vi "Frequency_sweep_measureXandY_w_2w_3w_MFLI_PK_v4.0.vi"() -> ()   [LabVIEW 2016]
uses:
  Labview Drivers/MFLI/LabOneLabVIEW-22.02.26577/LabOneLabVIEW-22.02.26577/Zurich Instruments LabOne/Public/Data/ziTypeDemodSampleSingle.ctl
  Labview Drivers/MFLI/LabOneLabVIEW-22.02.26577/LabOneLabVIEW-22.02.26577/Zurich Instruments LabOne/Public/Configure/ziSetValueDouble.vi
  Labview Drivers/MFLI/LabOneLabVIEW-22.02.26577/LabOneLabVIEW-22.02.26577/Zurich Instruments LabOne/Public/Configure/ziGetValueDemodSampleEx.vi
  Labview Drivers/MFLI/LabOneLabVIEW-22.02.26577/LabOneLabVIEW-22.02.26577/Zurich Instruments LabOne/Zurich Instruments LabOne.lvlib
panel:
  in  "Tab Control":T1(tab)=enum."Vy"
  out "Vx_w vs  Frequency":cluster{dbl, "Field Reading":dbl}[](graph)=[{2.1337108522522826e-07, "Field Reading"=1.0007121497539348e-06}, {2.0018204953851064e-08, "Field Reading"=1.0969598663661376e-07}, {3.474074033482476e-08, "Field Reading"=1.9016075130631681e-07}, {5.6400419155691035e-08, "Field Reading"=2.706780203266455e-07}, {7.134741663483111e-08, "Field Reading"=3.625194153695155e-07}, {8.711957733763268e-08, "Field Reading"=4.6186456260881066e-07}, {1.039613386460647e-07, "Field Reading"=5.541771498802743e-07}, {1.290159481540569e-07, "Field Reading"=6.517488283090827e-07}, {1.442006622421336e-07, "Field Reading"=7.441421685111633e-07}, {1.6579779771841864e-07, "Field Reading"=8.4200282004452e-07}, {1.7667431320194624e-07, "Field Reading"=9.371894272094692e-07}, {2.0346799660082097e-07, "Field Reading"=1.0346819690568719e-06}, {2.1275449478314156e-07, "Field Reading"=1.1273455634288892e-06}, {2.2792303722372882e-07, "Field Reading"=1.2246113813938451e-06}, {2.506226161778463e-07, "Field Reading"=1.3169699353558023e-06}, {2.6686786096204173e-07, "Field Reading"=1.4106741902497636e-06}, {2.979630377408132e-07, "Field Reading"=1.5068897992871093e-06}, {3.1162936250255217e-07, "Field Reading"=1.6013785409354697e-06}, {3.2854904168138843e-07, "Field Reading"=1.7007967107121696e-06}, {3.4501678279448686e-07, "Field Reading"=1.7932741209540488e-06}, {3.5732655253185603e-07, "Field Reading"=1.891133061059139e-06}, {3.7678513716337806e-07, "Field Reading"=1.9837632139333797e-06}, {3.8857693765173823e-07, "Field Reading"=2.078638757139878e-06}, {4.070455630330932e-07, "Field Reading"=2.1777621608691614e-06}, {4.3651006057087547e-07, "Field Reading"=2.270487653250022e-06}, {4.535609885287045e-07, "Field Reading"=2.364817703267964e-06}, {4.800092323465329e-07, "Field Reading"=2.4630513126122318e-06}, {4.872172260420143e-07, "Field Reading"=2.560612214294704e-06}, {5.029105394973937e-07, "Field Reading"=2.653407522930296e-06}, {5.207137968885614e-07, "Field Reading"=2.7508846993110185e-06}, {5.449974912672081e-07, "Field Reading"=2.8437164663468094e-06}, {5.549097834910874e-07, "Field Reading"=2.941117576580943e-06}, {5.789147944756835e-07, "Field Reading"=3.0334756142859178e-06}, {5.940331669154695e-07, "Field Reading"=3.130923358288321e-06}, {6.192662248173834e-07, "Field Reading"=3.223457045619671e-06}, {6.338859460756282e-07, "Field Reading"=3.3210140787077685e-06}, {6.617730672082958e-07, "Field Reading"=3.4134337904467758e-06}, {6.708744764433933e-07, "Field Reading"=3.511218639909905e-06}, {6.876034184888421e-07, "Field Reading"=3.6064791588715936e-06}, {7.081705825683568e-07, "Field Reading"=3.704194984998823e-06}, {7.341349902267621e-07, "Field Reading"=3.796795088130521e-06}, {7.500412173627324e-07, "Field Reading"=3.894221622472711e-06}, {7.635282212201655e-07, "Field Reading"=3.986359362120525e-06}, {7.839559208505005e-07, "Field Reading"=4.084105589459172e-06}, {7.991337007295971e-07, "Field Reading"=4.176440151889332e-06}, {8.175550663233945e-07, "Field Reading"=4.274041338897146e-06}, {8.360511976155764e-07, "Field Reading"=4.366718612721536e-06}, {8.595654269642977e-07, "Field Reading"=4.46481586459238e-06}, {8.846044621269243e-07, "Field Reading"=4.559710869350914e-06}, {8.902214589762566e-07, "Field Reading"=4.6535858762473605e-06}, {9.13930972707384e-07, "Field Reading"=4.751211544539011e-06}, {9.218629476317926e-07, "Field Reading"=4.843674806906942e-06}, {9.389346568153207e-07, "Field Reading"=4.94148963023105e-06}, {9.661788530141893e-07, "Field Reading"=5.0340339305698605e-06}, {9.734275114489362e-07, "Field Reading"=5.134274890899915e-06}, {9.91273930192609e-07, "Field Reading"=5.227194198108034e-06}, {1.0062090937222443e-06, "Field Reading"=5.324543514118811e-06}, {1.0324830232331714e-06, "Field Reading"=5.417068558459935e-06}, {1.0500453704719826e-06, "Field Reading"=5.514414049876445e-06}, {1.0818020141498576e-06, "Field Reading"=5.606738838727315e-06}, {1.0919981214621985e-06, "Field Reading"=5.943499955969014e-06}, {1.1041062115858416e-06, "Field Reading"=5.802825671371831e-06}, {1.12928896400331e-06, "Field Reading"=5.8897635364887065e-06}, {1.1492595887607054e-06, "Field Reading"=5.986959246668246e-06}, {1.1525838773614565e-06, "Field Reading"=6.079112281920131e-06}, {1.1732006667255544e-06, "Field Reading"=6.176765549637453e-06}, {1.193444625294635e-06, "Field Reading"=6.2693583656248445e-06}, {1.2101538188023656e-06, "Field Reading"=6.369277338631168e-06}, {1.2318147585414787e-06, "Field Reading"=6.462177680852612e-06}, {1.2413491771177379e-06, "Field Reading"=6.554239754143973e-06}, {1.2731631837142253e-06, "Field Reading"=6.653541226069562e-06}, {1.2825564782833625e-06, "Field Reading"=6.7454110623267924e-06}, {1.2992348301055137e-06, "Field Reading"=6.843115368447837e-06}, {1.316693256967963e-06, "Field Reading"=6.935702965257668e-06}, {1.343852132299077e-06, "Field Reading"=7.033596304342718e-06}, {0.0003223256295561193, "Field Reading"=7.130369502789653e-06}, {0.0010682796466779994, "Field Reading"=7.237712618778445e-06}, {0.0011012721847992696, "Field Reading"=7.315133567183911e-06}, {0.0011336841810168491, "Field Reading"=7.4123545054478695e-06}, {0.0011614058556892847, "Field Reading"=7.504304430827025e-06}, {0.001182885890671154, "Field Reading"=7.602366955750201e-06}, {0.001200897535521615, "Field Reading"=7.69976061587441e-06}, {0.00121594401470624, "Field Reading"=7.792677109208386e-06}, {0.0012308027651267619, "Field Reading"=7.886128685028496e-06}, {0.0012456418637471253, "Field Reading"=7.983615236672288e-06}, {0.001257564969772003, "Field Reading"=8.075760842161778e-06}, {0.0012690336996615858, "Field Reading"=8.170723157183957e-06}, {0.0012814644345765262, "Field Reading"=8.268995175290895e-06}, {0.0012910253378675095, "Field Reading"=8.363131378141633e-06}, {0.001301444806581894, "Field Reading"=8.45644533427298e-06}, {0.0013106148752890106, "Field Reading"=8.551458283635111e-06}, {0.0013201336522581891, "Field Reading"=8.65161959339898e-06}, {0.0013282012490195363, "Field Reading"=8.74416723601607e-06}, {0.0013370451945670784, "Field Reading"=8.841765835802203e-06}, {0.001345475691336453, "Field Reading"=8.933978266213217e-06}, {0.0013541642420234728, "Field Reading"=9.031643266856203e-06}, {0.0013602243952778926, "Field Reading"=9.123705087732138e-06}, {0.0013678078924535615, "Field Reading"=9.221510724442928e-06}, {0.0013749931650039048, "Field Reading"=9.319154251910434e-06}, {0.0013817418853904447, "Field Reading"=9.409423170522308e-06}, {0.0013877620940512577, "Field Reading"=9.50720467327743e-06}, {0.0013893900209027232, "Field Reading"=9.522740574798281e-06}, {0.0013841293323999348, "Field Reading"=9.444358568387913e-06}, {0.0013770955503089543, "Field Reading"=9.34786117205707e-06}, {0.0013707463881856257, "Field Reading"=9.255459479065146e-06}, {0.0013638010752030354, "Field Reading"=9.157506360964617e-06}, {0.001356127430849226, "Field Reading"=9.065389480276688e-06}, {0.0013481807501391138, "Field Reading"=8.967105386552946e-06}, {0.0013407950243109453, "Field Reading"=8.872574329619889e-06}, {0.0013327879049762552, "Field Reading"=8.780745564878272e-06}, {0.0013239176518001648, "Field Reading"=8.686977265427215e-06}, {0.0013146578852826479, "Field Reading"=8.586299385882446e-06}, {0.0013048672888862206, "Field Reading"=8.493635331032656e-06}, {0.0012950842712132512, "Field Reading"=8.395823484571033e-06}, {0.0012855051336405129, "Field Reading"=8.303455420153361e-06}, {0.001274818349601112, "Field Reading"=8.209679742685101e-06}, {0.0012618971608759537, "Field Reading"=8.109946125115199e-06}, {0.0012494525821266837, "Field Reading"=8.017364894823338e-06}, {0.001235685913286103, "Field Reading"=7.919657723881713e-06}, {0.0012216877307261714, "Field Reading"=7.824897358413329e-06}, {0.0012037516065472435, "Field Reading"=7.727435253164315e-06}, {0.0011875344677767074, "Field Reading"=7.634970945479442e-06}, {0.0011690885694813937, "Field Reading"=7.537773175917453e-06}, {0.001143867923079635, "Field Reading"=7.445625913634191e-06}, {0.0011139726709101221, "Field Reading"=7.348337041113834e-06}, {0.0010813147907609588, "Field Reading"=7.255852572757193e-06}, {0.0008158901453383064, "Field Reading"=7.15654215348316e-06}, {0.00014586885402730632, "Field Reading"=7.065078532967033e-06}, {6.672313176192101e-06, "Field Reading"=6.97131792702715e-06}, {1.311378694927265e-06, "Field Reading"=6.8592321760864306e-06}, {1.318127585000335e-06, "Field Reading"=6.78165201436255e-06}, {1.2916070805813707e-06, "Field Reading"=6.684382236814962e-06}, {1.2637872492482735e-06, "Field Reading"=6.591615618281428e-06}, {1.2510857193087697e-06, "Field Reading"=6.49373019741343e-06}, {1.2409566576000475e-06, "Field Reading"=6.399307801408899e-06}, {1.215389141425889e-06, "Field Reading"=6.305912312991265e-06}, {1.1948309642776338e-06, "Field Reading"=6.211147873874382e-06}, {1.1729714746286896e-06, "Field Reading"=6.112674813622632e-06}, {1.1526746179431637e-06, "Field Reading"=6.015256707500007e-06}]
  out "Vy_w vs Frequency":cluster{dbl, "Field Reading":dbl}[](graph)=[{2.1337108522522826e-07, "Field Reading"=1.0007121497539348e-06}, {2.0018204953851064e-08, "Field Reading"=1.0969598663661376e-07}, {3.474074033482476e-08, "Field Reading"=1.9016075130631681e-07}, {5.6400419155691035e-08, "Field Reading"=2.706780203266455e-07}, {7.134741663483111e-08, "Field Reading"=3.625194153695155e-07}, {8.711957733763268e-08, "Field Reading"=4.6186456260881066e-07}, {1.039613386460647e-07, "Field Reading"=5.541771498802743e-07}, {1.290159481540569e-07, "Field Reading"=6.517488283090827e-07}, {1.442006622421336e-07, "Field Reading"=7.441421685111633e-07}, {1.6579779771841864e-07, "Field Reading"=8.4200282004452e-07}, {1.7667431320194624e-07, "Field Reading"=9.371894272094692e-07}, {2.0346799660082097e-07, "Field Reading"=1.0346819690568719e-06}, {2.1275449478314156e-07, "Field Reading"=1.1273455634288892e-06}, {2.2792303722372882e-07, "Field Reading"=1.2246113813938451e-06}, {2.506226161778463e-07, "Field Reading"=1.3169699353558023e-06}, {2.6686786096204173e-07, "Field Reading"=1.4106741902497636e-06}, {2.979630377408132e-07, "Field Reading"=1.5068897992871093e-06}, {3.1162936250255217e-07, "Field Reading"=1.6013785409354697e-06}, {3.2854904168138843e-07, "Field Reading"=1.7007967107121696e-06}, {3.4501678279448686e-07, "Field Reading"=1.7932741209540488e-06}, {3.5732655253185603e-07, "Field Reading"=1.891133061059139e-06}, {3.7678513716337806e-07, "Field Reading"=1.9837632139333797e-06}, {3.8857693765173823e-07, "Field Reading"=2.078638757139878e-06}, {4.070455630330932e-07, "Field Reading"=2.1777621608691614e-06}, {4.3651006057087547e-07, "Field Reading"=2.270487653250022e-06}, {4.535609885287045e-07, "Field Reading"=2.364817703267964e-06}, {4.800092323465329e-07, "Field Reading"=2.4630513126122318e-06}, {4.872172260420143e-07, "Field Reading"=2.560612214294704e-06}, {5.029105394973937e-07, "Field Reading"=2.653407522930296e-06}, {5.207137968885614e-07, "Field Reading"=2.7508846993110185e-06}, {5.449974912672081e-07, "Field Reading"=2.8437164663468094e-06}, {5.549097834910874e-07, "Field Reading"=2.941117576580943e-06}, {5.789147944756835e-07, "Field Reading"=3.0334756142859178e-06}, {5.940331669154695e-07, "Field Reading"=3.130923358288321e-06}, {6.192662248173834e-07, "Field Reading"=3.223457045619671e-06}, {6.338859460756282e-07, "Field Reading"=3.3210140787077685e-06}, {6.617730672082958e-07, "Field Reading"=3.4134337904467758e-06}, {6.708744764433933e-07, "Field Reading"=3.511218639909905e-06}, {6.876034184888421e-07, "Field Reading"=3.6064791588715936e-06}, {7.081705825683568e-07, "Field Reading"=3.704194984998823e-06}, {7.341349902267621e-07, "Field Reading"=3.796795088130521e-06}, {7.500412173627324e-07, "Field Reading"=3.894221622472711e-06}, {7.635282212201655e-07, "Field Reading"=3.986359362120525e-06}, {7.839559208505005e-07, "Field Reading"=4.084105589459172e-06}, {7.991337007295971e-07, "Field Reading"=4.176440151889332e-06}, {8.175550663233945e-07, "Field Reading"=4.274041338897146e-06}, {8.360511976155764e-07, "Field Reading"=4.366718612721536e-06}, {8.595654269642977e-07, "Field Reading"=4.46481586459238e-06}, {8.846044621269243e-07, "Field Reading"=4.559710869350914e-06}, {8.902214589762566e-07, "Field Reading"=4.6535858762473605e-06}, {9.13930972707384e-07, "Field Reading"=4.751211544539011e-06}, {9.218629476317926e-07, "Field Reading"=4.843674806906942e-06}, {9.389346568153207e-07, "Field Reading"=4.94148963023105e-06}, {9.661788530141893e-07, "Field Reading"=5.0340339305698605e-06}, {9.734275114489362e-07, "Field Reading"=5.134274890899915e-06}, {9.91273930192609e-07, "Field Reading"=5.227194198108034e-06}, {1.0062090937222443e-06, "Field Reading"=5.324543514118811e-06}, {1.0324830232331714e-06, "Field Reading"=5.417068558459935e-06}, {1.0500453704719826e-06, "Field Reading"=5.514414049876445e-06}, {1.0818020141498576e-06, "Field Reading"=5.606738838727315e-06}, {1.0919981214621985e-06, "Field Reading"=5.943499955969014e-06}, {1.1041062115858416e-06, "Field Reading"=5.802825671371831e-06}, {1.12928896400331e-06, "Field Reading"=5.8897635364887065e-06}, {1.1492595887607054e-06, "Field Reading"=5.986959246668246e-06}, {1.1525838773614565e-06, "Field Reading"=6.079112281920131e-06}, {1.1732006667255544e-06, "Field Reading"=6.176765549637453e-06}, {1.193444625294635e-06, "Field Reading"=6.2693583656248445e-06}, {1.2101538188023656e-06, "Field Reading"=6.369277338631168e-06}, {1.2318147585414787e-06, "Field Reading"=6.462177680852612e-06}, {1.2413491771177379e-06, "Field Reading"=6.554239754143973e-06}, {1.2731631837142253e-06, "Field Reading"=6.653541226069562e-06}, {1.2825564782833625e-06, "Field Reading"=6.7454110623267924e-06}, {1.2992348301055137e-06, "Field Reading"=6.843115368447837e-06}, {1.316693256967963e-06, "Field Reading"=6.935702965257668e-06}, {1.343852132299077e-06, "Field Reading"=7.033596304342718e-06}, {0.0003223256295561193, "Field Reading"=7.130369502789653e-06}, {0.0010682796466779994, "Field Reading"=7.237712618778445e-06}, {0.0011012721847992696, "Field Reading"=7.315133567183911e-06}, {0.0011336841810168491, "Field Reading"=7.4123545054478695e-06}, {0.0011614058556892847, "Field Reading"=7.504304430827025e-06}, {0.001182885890671154, "Field Reading"=7.602366955750201e-06}, {0.001200897535521615, "Field Reading"=7.69976061587441e-06}, {0.00121594401470624, "Field Reading"=7.792677109208386e-06}, {0.0012308027651267619, "Field Reading"=7.886128685028496e-06}, {0.0012456418637471253, "Field Reading"=7.983615236672288e-06}, {0.001257564969772003, "Field Reading"=8.075760842161778e-06}, {0.0012690336996615858, "Field Reading"=8.170723157183957e-06}, {0.0012814644345765262, "Field Reading"=8.268995175290895e-06}, {0.0012910253378675095, "Field Reading"=8.363131378141633e-06}, {0.001301444806581894, "Field Reading"=8.45644533427298e-06}, {0.0013106148752890106, "Field Reading"=8.551458283635111e-06}, {0.0013201336522581891, "Field Reading"=8.65161959339898e-06}, {0.0013282012490195363, "Field Reading"=8.74416723601607e-06}, {0.0013370451945670784, "Field Reading"=8.841765835802203e-06}, {0.001345475691336453, "Field Reading"=8.933978266213217e-06}, {0.0013541642420234728, "Field Reading"=9.031643266856203e-06}, {0.0013602243952778926, "Field Reading"=9.123705087732138e-06}, {0.0013678078924535615, "Field Reading"=9.221510724442928e-06}, {0.0013749931650039048, "Field Reading"=9.319154251910434e-06}, {0.0013817418853904447, "Field Reading"=9.409423170522308e-06}, {0.0013877620940512577, "Field Reading"=9.50720467327743e-06}, {0.0013893900209027232, "Field Reading"=9.522740574798281e-06}, {0.0013841293323999348, "Field Reading"=9.444358568387913e-06}, {0.0013770955503089543, "Field Reading"=9.34786117205707e-06}, {0.0013707463881856257, "Field Reading"=9.255459479065146e-06}, {0.0013638010752030354, "Field Reading"=9.157506360964617e-06}, {0.001356127430849226, "Field Reading"=9.065389480276688e-06}, {0.0013481807501391138, "Field Reading"=8.967105386552946e-06}, {0.0013407950243109453, "Field Reading"=8.872574329619889e-06}, {0.0013327879049762552, "Field Reading"=8.780745564878272e-06}, {0.0013239176518001648, "Field Reading"=8.686977265427215e-06}, {0.0013146578852826479, "Field Reading"=8.586299385882446e-06}, {0.0013048672888862206, "Field Reading"=8.493635331032656e-06}, {0.0012950842712132512, "Field Reading"=8.395823484571033e-06}, {0.0012855051336405129, "Field Reading"=8.303455420153361e-06}, {0.001274818349601112, "Field Reading"=8.209679742685101e-06}, {0.0012618971608759537, "Field Reading"=8.109946125115199e-06}, {0.0012494525821266837, "Field Reading"=8.017364894823338e-06}, {0.001235685913286103, "Field Reading"=7.919657723881713e-06}, {0.0012216877307261714, "Field Reading"=7.824897358413329e-06}, {0.0012037516065472435, "Field Reading"=7.727435253164315e-06}, {0.0011875344677767074, "Field Reading"=7.634970945479442e-06}, {0.0011690885694813937, "Field Reading"=7.537773175917453e-06}, {0.001143867923079635, "Field Reading"=7.445625913634191e-06}, {0.0011139726709101221, "Field Reading"=7.348337041113834e-06}, {0.0010813147907609588, "Field Reading"=7.255852572757193e-06}, {0.0008158901453383064, "Field Reading"=7.15654215348316e-06}, {0.00014586885402730632, "Field Reading"=7.065078532967033e-06}, {6.672313176192101e-06, "Field Reading"=6.97131792702715e-06}, {1.311378694927265e-06, "Field Reading"=6.8592321760864306e-06}, {1.318127585000335e-06, "Field Reading"=6.78165201436255e-06}, {1.2916070805813707e-06, "Field Reading"=6.684382236814962e-06}, {1.2637872492482735e-06, "Field Reading"=6.591615618281428e-06}, {1.2510857193087697e-06, "Field Reading"=6.49373019741343e-06}, {1.2409566576000475e-06, "Field Reading"=6.399307801408899e-06}, {1.215389141425889e-06, "Field Reading"=6.305912312991265e-06}, {1.1948309642776338e-06, "Field Reading"=6.211147873874382e-06}, {1.1729714746286896e-06, "Field Reading"=6.112674813622632e-06}, {1.1526746179431637e-06, "Field Reading"=6.015256707500007e-06}]
  out "Inductive reactance vs  Frequency":cluster{dbl, "Field Reading":dbl}[](graph)=[{2.1337108522522826e-07, "Field Reading"=1.0007121497539348e-06}, {2.0018204953851064e-08, "Field Reading"=1.0969598663661376e-07}, {3.474074033482476e-08, "Field Reading"=1.9016075130631681e-07}, {5.6400419155691035e-08, "Field Reading"=2.706780203266455e-07}, {7.134741663483111e-08, "Field Reading"=3.625194153695155e-07}, {8.711957733763268e-08, "Field Reading"=4.6186456260881066e-07}, {1.039613386460647e-07, "Field Reading"=5.541771498802743e-07}, {1.290159481540569e-07, "Field Reading"=6.517488283090827e-07}, {1.442006622421336e-07, "Field Reading"=7.441421685111633e-07}, {1.6579779771841864e-07, "Field Reading"=8.4200282004452e-07}, {1.7667431320194624e-07, "Field Reading"=9.371894272094692e-07}, {2.0346799660082097e-07, "Field Reading"=1.0346819690568719e-06}, {2.1275449478314156e-07, "Field Reading"=1.1273455634288892e-06}, {2.2792303722372882e-07, "Field Reading"=1.2246113813938451e-06}, {2.506226161778463e-07, "Field Reading"=1.3169699353558023e-06}, {2.6686786096204173e-07, "Field Reading"=1.4106741902497636e-06}, {2.979630377408132e-07, "Field Reading"=1.5068897992871093e-06}, {3.1162936250255217e-07, "Field Reading"=1.6013785409354697e-06}, {3.2854904168138843e-07, "Field Reading"=1.7007967107121696e-06}, {3.4501678279448686e-07, "Field Reading"=1.7932741209540488e-06}, {3.5732655253185603e-07, "Field Reading"=1.891133061059139e-06}, {3.7678513716337806e-07, "Field Reading"=1.9837632139333797e-06}, {3.8857693765173823e-07, "Field Reading"=2.078638757139878e-06}, {4.070455630330932e-07, "Field Reading"=2.1777621608691614e-06}, {4.3651006057087547e-07, "Field Reading"=2.270487653250022e-06}, {4.535609885287045e-07, "Field Reading"=2.364817703267964e-06}, {4.800092323465329e-07, "Field Reading"=2.4630513126122318e-06}, {4.872172260420143e-07, "Field Reading"=2.560612214294704e-06}, {5.029105394973937e-07, "Field Reading"=2.653407522930296e-06}, {5.207137968885614e-07, "Field Reading"=2.7508846993110185e-06}, {5.449974912672081e-07, "Field Reading"=2.8437164663468094e-06}, {5.549097834910874e-07, "Field Reading"=2.941117576580943e-06}, {5.789147944756835e-07, "Field Reading"=3.0334756142859178e-06}, {5.940331669154695e-07, "Field Reading"=3.130923358288321e-06}, {6.192662248173834e-07, "Field Reading"=3.223457045619671e-06}, {6.338859460756282e-07, "Field Reading"=3.3210140787077685e-06}, {6.617730672082958e-07, "Field Reading"=3.4134337904467758e-06}, {6.708744764433933e-07, "Field Reading"=3.511218639909905e-06}, {6.876034184888421e-07, "Field Reading"=3.6064791588715936e-06}, {7.081705825683568e-07, "Field Reading"=3.704194984998823e-06}, {7.341349902267621e-07, "Field Reading"=3.796795088130521e-06}, {7.500412173627324e-07, "Field Reading"=3.894221622472711e-06}, {7.635282212201655e-07, "Field Reading"=3.986359362120525e-06}, {7.839559208505005e-07, "Field Reading"=4.084105589459172e-06}, {7.991337007295971e-07, "Field Reading"=4.176440151889332e-06}, {8.175550663233945e-07, "Field Reading"=4.274041338897146e-06}, {8.360511976155764e-07, "Field Reading"=4.366718612721536e-06}, {8.595654269642977e-07, "Field Reading"=4.46481586459238e-06}, {8.846044621269243e-07, "Field Reading"=4.559710869350914e-06}, {8.902214589762566e-07, "Field Reading"=4.6535858762473605e-06}, {9.13930972707384e-07, "Field Reading"=4.751211544539011e-06}, {9.218629476317926e-07, "Field Reading"=4.843674806906942e-06}, {9.389346568153207e-07, "Field Reading"=4.94148963023105e-06}, {9.661788530141893e-07, "Field Reading"=5.0340339305698605e-06}, {9.734275114489362e-07, "Field Reading"=5.134274890899915e-06}, {9.91273930192609e-07, "Field Reading"=5.227194198108034e-06}, {1.0062090937222443e-06, "Field Reading"=5.324543514118811e-06}, {1.0324830232331714e-06, "Field Reading"=5.417068558459935e-06}, {1.0500453704719826e-06, "Field Reading"=5.514414049876445e-06}, {1.0818020141498576e-06, "Field Reading"=5.606738838727315e-06}, {1.0919981214621985e-06, "Field Reading"=5.943499955969014e-06}, {1.1041062115858416e-06, "Field Reading"=5.802825671371831e-06}, {1.12928896400331e-06, "Field Reading"=5.8897635364887065e-06}, {1.1492595887607054e-06, "Field Reading"=5.986959246668246e-06}, {1.1525838773614565e-06, "Field Reading"=6.079112281920131e-06}, {1.1732006667255544e-06, "Field Reading"=6.176765549637453e-06}, {1.193444625294635e-06, "Field Reading"=6.2693583656248445e-06}, {1.2101538188023656e-06, "Field Reading"=6.369277338631168e-06}, {1.2318147585414787e-06, "Field Reading"=6.462177680852612e-06}, {1.2413491771177379e-06, "Field Reading"=6.554239754143973e-06}, {1.2731631837142253e-06, "Field Reading"=6.653541226069562e-06}, {1.2825564782833625e-06, "Field Reading"=6.7454110623267924e-06}, {1.2992348301055137e-06, "Field Reading"=6.843115368447837e-06}, {1.316693256967963e-06, "Field Reading"=6.935702965257668e-06}, {1.343852132299077e-06, "Field Reading"=7.033596304342718e-06}, {0.0003223256295561193, "Field Reading"=7.130369502789653e-06}, {0.0010682796466779994, "Field Reading"=7.237712618778445e-06}, {0.0011012721847992696, "Field Reading"=7.315133567183911e-06}, {0.0011336841810168491, "Field Reading"=7.4123545054478695e-06}, {0.0011614058556892847, "Field Reading"=7.504304430827025e-06}, {0.001182885890671154, "Field Reading"=7.602366955750201e-06}, {0.001200897535521615, "Field Reading"=7.69976061587441e-06}, {0.00121594401470624, "Field Reading"=7.792677109208386e-06}, {0.0012308027651267619, "Field Reading"=7.886128685028496e-06}, {0.0012456418637471253, "Field Reading"=7.983615236672288e-06}, {0.001257564969772003, "Field Reading"=8.075760842161778e-06}, {0.0012690336996615858, "Field Reading"=8.170723157183957e-06}, {0.0012814644345765262, "Field Reading"=8.268995175290895e-06}, {0.0012910253378675095, "Field Reading"=8.363131378141633e-06}, {0.001301444806581894, "Field Reading"=8.45644533427298e-06}, {0.0013106148752890106, "Field Reading"=8.551458283635111e-06}, {0.0013201336522581891, "Field Reading"=8.65161959339898e-06}, {0.0013282012490195363, "Field Reading"=8.74416723601607e-06}, {0.0013370451945670784, "Field Reading"=8.841765835802203e-06}, {0.001345475691336453, "Field Reading"=8.933978266213217e-06}, {0.0013541642420234728, "Field Reading"=9.031643266856203e-06}, {0.0013602243952778926, "Field Reading"=9.123705087732138e-06}, {0.0013678078924535615, "Field Reading"=9.221510724442928e-06}, {0.0013749931650039048, "Field Reading"=9.319154251910434e-06}, {0.0013817418853904447, "Field Reading"=9.409423170522308e-06}, {0.0013877620940512577, "Field Reading"=9.50720467327743e-06}, {0.0013893900209027232, "Field Reading"=9.522740574798281e-06}, {0.0013841293323999348, "Field Reading"=9.444358568387913e-06}, {0.0013770955503089543, "Field Reading"=9.34786117205707e-06}, {0.0013707463881856257, "Field Reading"=9.255459479065146e-06}, {0.0013638010752030354, "Field Reading"=9.157506360964617e-06}, {0.001356127430849226, "Field Reading"=9.065389480276688e-06}, {0.0013481807501391138, "Field Reading"=8.967105386552946e-06}, {0.0013407950243109453, "Field Reading"=8.872574329619889e-06}, {0.0013327879049762552, "Field Reading"=8.780745564878272e-06}, {0.0013239176518001648, "Field Reading"=8.686977265427215e-06}, {0.0013146578852826479, "Field Reading"=8.586299385882446e-06}, {0.0013048672888862206, "Field Reading"=8.493635331032656e-06}, {0.0012950842712132512, "Field Reading"=8.395823484571033e-06}, {0.0012855051336405129, "Field Reading"=8.303455420153361e-06}, {0.001274818349601112, "Field Reading"=8.209679742685101e-06}, {0.0012618971608759537, "Field Reading"=8.109946125115199e-06}, {0.0012494525821266837, "Field Reading"=8.017364894823338e-06}, {0.001235685913286103, "Field Reading"=7.919657723881713e-06}, {0.0012216877307261714, "Field Reading"=7.824897358413329e-06}, {0.0012037516065472435, "Field Reading"=7.727435253164315e-06}, {0.0011875344677767074, "Field Reading"=7.634970945479442e-06}, {0.0011690885694813937, "Field Reading"=7.537773175917453e-06}, {0.001143867923079635, "Field Reading"=7.445625913634191e-06}, {0.0011139726709101221, "Field Reading"=7.348337041113834e-06}, {0.0010813147907609588, "Field Reading"=7.255852572757193e-06}, {0.0008158901453383064, "Field Reading"=7.15654215348316e-06}, {0.00014586885402730632, "Field Reading"=7.065078532967033e-06}, {6.672313176192101e-06, "Field Reading"=6.97131792702715e-06}, {1.311378694927265e-06, "Field Reading"=6.8592321760864306e-06}, {1.318127585000335e-06, "Field Reading"=6.78165201436255e-06}, {1.2916070805813707e-06, "Field Reading"=6.684382236814962e-06}, {1.2637872492482735e-06, "Field Reading"=6.591615618281428e-06}, {1.2510857193087697e-06, "Field Reading"=6.49373019741343e-06}, {1.2409566576000475e-06, "Field Reading"=6.399307801408899e-06}, {1.215389141425889e-06, "Field Reading"=6.305912312991265e-06}, {1.1948309642776338e-06, "Field Reading"=6.211147873874382e-06}, {1.1729714746286896e-06, "Field Reading"=6.112674813622632e-06}, {1.1526746179431637e-06, "Field Reading"=6.015256707500007e-06}]
  out "Inductance vs  Frequency":cluster{dbl, "Field Reading":dbl}[](graph)=[{2.1337108522522826e-07, "Field Reading"=1.0007121497539348e-06}, {2.0018204953851064e-08, "Field Reading"=1.0969598663661376e-07}, {3.474074033482476e-08, "Field Reading"=1.9016075130631681e-07}, {5.6400419155691035e-08, "Field Reading"=2.706780203266455e-07}, {7.134741663483111e-08, "Field Reading"=3.625194153695155e-07}, {8.711957733763268e-08, "Field Reading"=4.6186456260881066e-07}, {1.039613386460647e-07, "Field Reading"=5.541771498802743e-07}, {1.290159481540569e-07, "Field Reading"=6.517488283090827e-07}, {1.442006622421336e-07, "Field Reading"=7.441421685111633e-07}, {1.6579779771841864e-07, "Field Reading"=8.4200282004452e-07}, {1.7667431320194624e-07, "Field Reading"=9.371894272094692e-07}, {2.0346799660082097e-07, "Field Reading"=1.0346819690568719e-06}, {2.1275449478314156e-07, "Field Reading"=1.1273455634288892e-06}, {2.2792303722372882e-07, "Field Reading"=1.2246113813938451e-06}, {2.506226161778463e-07, "Field Reading"=1.3169699353558023e-06}, {2.6686786096204173e-07, "Field Reading"=1.4106741902497636e-06}, {2.979630377408132e-07, "Field Reading"=1.5068897992871093e-06}, {3.1162936250255217e-07, "Field Reading"=1.6013785409354697e-06}, {3.2854904168138843e-07, "Field Reading"=1.7007967107121696e-06}, {3.4501678279448686e-07, "Field Reading"=1.7932741209540488e-06}, {3.5732655253185603e-07, "Field Reading"=1.891133061059139e-06}, {3.7678513716337806e-07, "Field Reading"=1.9837632139333797e-06}, {3.8857693765173823e-07, "Field Reading"=2.078638757139878e-06}, {4.070455630330932e-07, "Field Reading"=2.1777621608691614e-06}, {4.3651006057087547e-07, "Field Reading"=2.270487653250022e-06}, {4.535609885287045e-07, "Field Reading"=2.364817703267964e-06}, {4.800092323465329e-07, "Field Reading"=2.4630513126122318e-06}, {4.872172260420143e-07, "Field Reading"=2.560612214294704e-06}, {5.029105394973937e-07, "Field Reading"=2.653407522930296e-06}, {5.207137968885614e-07, "Field Reading"=2.7508846993110185e-06}, {5.449974912672081e-07, "Field Reading"=2.8437164663468094e-06}, {5.549097834910874e-07, "Field Reading"=2.941117576580943e-06}, {5.789147944756835e-07, "Field Reading"=3.0334756142859178e-06}, {5.940331669154695e-07, "Field Reading"=3.130923358288321e-06}, {6.192662248173834e-07, "Field Reading"=3.223457045619671e-06}, {6.338859460756282e-07, "Field Reading"=3.3210140787077685e-06}, {6.617730672082958e-07, "Field Reading"=3.4134337904467758e-06}, {6.708744764433933e-07, "Field Reading"=3.511218639909905e-06}, {6.876034184888421e-07, "Field Reading"=3.6064791588715936e-06}, {7.081705825683568e-07, "Field Reading"=3.704194984998823e-06}, {7.341349902267621e-07, "Field Reading"=3.796795088130521e-06}, {7.500412173627324e-07, "Field Reading"=3.894221622472711e-06}, {7.635282212201655e-07, "Field Reading"=3.986359362120525e-06}, {7.839559208505005e-07, "Field Reading"=4.084105589459172e-06}, {7.991337007295971e-07, "Field Reading"=4.176440151889332e-06}, {8.175550663233945e-07, "Field Reading"=4.274041338897146e-06}, {8.360511976155764e-07, "Field Reading"=4.366718612721536e-06}, {8.595654269642977e-07, "Field Reading"=4.46481586459238e-06}, {8.846044621269243e-07, "Field Reading"=4.559710869350914e-06}, {8.902214589762566e-07, "Field Reading"=4.6535858762473605e-06}, {9.13930972707384e-07, "Field Reading"=4.751211544539011e-06}, {9.218629476317926e-07, "Field Reading"=4.843674806906942e-06}, {9.389346568153207e-07, "Field Reading"=4.94148963023105e-06}, {9.661788530141893e-07, "Field Reading"=5.0340339305698605e-06}, {9.734275114489362e-07, "Field Reading"=5.134274890899915e-06}, {9.91273930192609e-07, "Field Reading"=5.227194198108034e-06}, {1.0062090937222443e-06, "Field Reading"=5.324543514118811e-06}, {1.0324830232331714e-06, "Field Reading"=5.417068558459935e-06}, {1.0500453704719826e-06, "Field Reading"=5.514414049876445e-06}, {1.0818020141498576e-06, "Field Reading"=5.606738838727315e-06}, {1.0919981214621985e-06, "Field Reading"=5.943499955969014e-06}, {1.1041062115858416e-06, "Field Reading"=5.802825671371831e-06}, {1.12928896400331e-06, "Field Reading"=5.8897635364887065e-06}, {1.1492595887607054e-06, "Field Reading"=5.986959246668246e-06}, {1.1525838773614565e-06, "Field Reading"=6.079112281920131e-06}, {1.1732006667255544e-06, "Field Reading"=6.176765549637453e-06}, {1.193444625294635e-06, "Field Reading"=6.2693583656248445e-06}, {1.2101538188023656e-06, "Field Reading"=6.369277338631168e-06}, {1.2318147585414787e-06, "Field Reading"=6.462177680852612e-06}, {1.2413491771177379e-06, "Field Reading"=6.554239754143973e-06}, {1.2731631837142253e-06, "Field Reading"=6.653541226069562e-06}, {1.2825564782833625e-06, "Field Reading"=6.7454110623267924e-06}, {1.2992348301055137e-06, "Field Reading"=6.843115368447837e-06}, {1.316693256967963e-06, "Field Reading"=6.935702965257668e-06}, {1.343852132299077e-06, "Field Reading"=7.033596304342718e-06}, {0.0003223256295561193, "Field Reading"=7.130369502789653e-06}, {0.0010682796466779994, "Field Reading"=7.237712618778445e-06}, {0.0011012721847992696, "Field Reading"=7.315133567183911e-06}, {0.0011336841810168491, "Field Reading"=7.4123545054478695e-06}, {0.0011614058556892847, "Field Reading"=7.504304430827025e-06}, {0.001182885890671154, "Field Reading"=7.602366955750201e-06}, {0.001200897535521615, "Field Reading"=7.69976061587441e-06}, {0.00121594401470624, "Field Reading"=7.792677109208386e-06}, {0.0012308027651267619, "Field Reading"=7.886128685028496e-06}, {0.0012456418637471253, "Field Reading"=7.983615236672288e-06}, {0.001257564969772003, "Field Reading"=8.075760842161778e-06}, {0.0012690336996615858, "Field Reading"=8.170723157183957e-06}, {0.0012814644345765262, "Field Reading"=8.268995175290895e-06}, {0.0012910253378675095, "Field Reading"=8.363131378141633e-06}, {0.001301444806581894, "Field Reading"=8.45644533427298e-06}, {0.0013106148752890106, "Field Reading"=8.551458283635111e-06}, {0.0013201336522581891, "Field Reading"=8.65161959339898e-06}, {0.0013282012490195363, "Field Reading"=8.74416723601607e-06}, {0.0013370451945670784, "Field Reading"=8.841765835802203e-06}, {0.001345475691336453, "Field Reading"=8.933978266213217e-06}, {0.0013541642420234728, "Field Reading"=9.031643266856203e-06}, {0.0013602243952778926, "Field Reading"=9.123705087732138e-06}, {0.0013678078924535615, "Field Reading"=9.221510724442928e-06}, {0.0013749931650039048, "Field Reading"=9.319154251910434e-06}, {0.0013817418853904447, "Field Reading"=9.409423170522308e-06}, {0.0013877620940512577, "Field Reading"=9.50720467327743e-06}, {0.0013893900209027232, "Field Reading"=9.522740574798281e-06}, {0.0013841293323999348, "Field Reading"=9.444358568387913e-06}, {0.0013770955503089543, "Field Reading"=9.34786117205707e-06}, {0.0013707463881856257, "Field Reading"=9.255459479065146e-06}, {0.0013638010752030354, "Field Reading"=9.157506360964617e-06}, {0.001356127430849226, "Field Reading"=9.065389480276688e-06}, {0.0013481807501391138, "Field Reading"=8.967105386552946e-06}, {0.0013407950243109453, "Field Reading"=8.872574329619889e-06}, {0.0013327879049762552, "Field Reading"=8.780745564878272e-06}, {0.0013239176518001648, "Field Reading"=8.686977265427215e-06}, {0.0013146578852826479, "Field Reading"=8.586299385882446e-06}, {0.0013048672888862206, "Field Reading"=8.493635331032656e-06}, {0.0012950842712132512, "Field Reading"=8.395823484571033e-06}, {0.0012855051336405129, "Field Reading"=8.303455420153361e-06}, {0.001274818349601112, "Field Reading"=8.209679742685101e-06}, {0.0012618971608759537, "Field Reading"=8.109946125115199e-06}, {0.0012494525821266837, "Field Reading"=8.017364894823338e-06}, {0.001235685913286103, "Field Reading"=7.919657723881713e-06}, {0.0012216877307261714, "Field Reading"=7.824897358413329e-06}, {0.0012037516065472435, "Field Reading"=7.727435253164315e-06}, {0.0011875344677767074, "Field Reading"=7.634970945479442e-06}, {0.0011690885694813937, "Field Reading"=7.537773175917453e-06}, {0.001143867923079635, "Field Reading"=7.445625913634191e-06}, {0.0011139726709101221, "Field Reading"=7.348337041113834e-06}, {0.0010813147907609588, "Field Reading"=7.255852572757193e-06}, {0.0008158901453383064, "Field Reading"=7.15654215348316e-06}, {0.00014586885402730632, "Field Reading"=7.065078532967033e-06}, {6.672313176192101e-06, "Field Reading"=6.97131792702715e-06}, {1.311378694927265e-06, "Field Reading"=6.8592321760864306e-06}, {1.318127585000335e-06, "Field Reading"=6.78165201436255e-06}, {1.2916070805813707e-06, "Field Reading"=6.684382236814962e-06}, {1.2637872492482735e-06, "Field Reading"=6.591615618281428e-06}, {1.2510857193087697e-06, "Field Reading"=6.49373019741343e-06}, {1.2409566576000475e-06, "Field Reading"=6.399307801408899e-06}, {1.215389141425889e-06, "Field Reading"=6.305912312991265e-06}, {1.1948309642776338e-06, "Field Reading"=6.211147873874382e-06}, {1.1729714746286896e-06, "Field Reading"=6.112674813622632e-06}, {1.1526746179431637e-06, "Field Reading"=6.015256707500007e-06}]
  out "Inductance (H)":dbl format="%#_13g"
  out "Inductive reactance":dbl format="%#_13g"
  out "Oscillator Frequency (Hz)":dbl format="%#_13g"
  in  "Autophase?":bool
  in  "Autorange?":bool
  in  "Number averaging":i32=10
  out "Vy_3w (V)":dbl=40.57455732074348 format="%#_13g"
  out "Demod Sample Out 4":T2={"Timestamps (ticks)"=217071887690750, "X (Vrms)"=8.75456933556226e-07, "Y (Vrms)"=7.498226005787958e-07, "Osc Phase (deg)"=5.4774618983426535, "Freq (Hz)"=7.919000069023241, "DIO"=0, "AuxIn0 (V)"=-0.001673382503213361, "AuxIn1 (V)"=-0.0006673162570223212, "Trigger"=512}
  out "Vx_3w (V)":dbl=1.1526746179431637e-06
  out "Vy_2w (V)":dbl=40.57455732074348 format="%#_13g"
  out "Demod Sample Out 3":T2={"Timestamps (ticks)"=217071887690750, "X (Vrms)"=8.75456933556226e-07, "Y (Vrms)"=7.498226005787958e-07, "Osc Phase (deg)"=5.4774618983426535, "Freq (Hz)"=7.919000069023241, "DIO"=0, "AuxIn0 (V)"=-0.001673382503213361, "AuxIn1 (V)"=-0.0006673162570223212, "Trigger"=512}
  out "Vx_2w (V)":dbl=1.1526746179431637e-06
  out "Iy_w (A)":dbl=-16.59997463839791 format="%#_13g"
  out "Vy_w (V)":dbl=40.57455732074348 format="%#_13g"
  out "Time(s)":dbl=185.322 format="%#_13g"
  out "Demod Sample Out 2":T2={"Timestamps (ticks)"=217071890701310, "X (Vrms)"=5.764492493379272e-06, "Y (Vrms)"=-1.7187028687058897e-06, "Osc Phase (deg)"=1.9746167692057917, "Freq (Hz)"=7.919000069023241, "DIO"=0, "AuxIn0 (V)"=-0.0006693530012853444, "AuxIn1 (V)"=0.0, "Trigger"=256}
  out "Demod Sample Out":T2={"Timestamps (ticks)"=217071887690750, "X (Vrms)"=8.75456933556226e-07, "Y (Vrms)"=7.498226005787958e-07, "Osc Phase (deg)"=5.4774618983426535, "Freq (Hz)"=7.919000069023241, "DIO"=0, "AuxIn0 (V)"=-0.001673382503213361, "AuxIn1 (V)"=-0.0006673162570223212, "Trigger"=512}
  in  "MFLI Current source/Voltage reader":string="DEV4382"
  out "Ix_w (A)":dbl=6.015256707500007e-06
  out "Vx_w (V)":dbl=1.1526746179431637e-06
  in  "Folder":path=path "D:/Pranava/Data/Inductance measurement test"
  in  "wait (ms) [Should be > TC]":u32=1000
  out "data":dbl[](array[numeric])=[1.1526746179431637e-06, 6.015256707500007e-06, 3.1500000000000066, 184.117, 40.57455732074348, -16.59997463839791]
  in  "Step":dbl[](array[numeric])=[10.0] min=-3000.0 max=3000.0 format="%.1e"
  in  "To":dbl[](array[numeric])=[10000.0] min=-3000.0 max=3000.0 format="%.1e"
  in  "From":dbl[](array[numeric])=[7.0] min=-3000.0 max=3000.0 format="%.1e"
  in  "file name":string="002_1uH_standard_300K_test"
  out "File path":path=path "D:/Heng/Nb3Br8_JJ/Sb.3_NBVJ01/20210115/002_NBVJ01_IV(8mK)_I16_R34_ac(13.3337Hz).dat"
  # ".dat"
  # "Set MFLI Oscillator Frequency (Hz)"
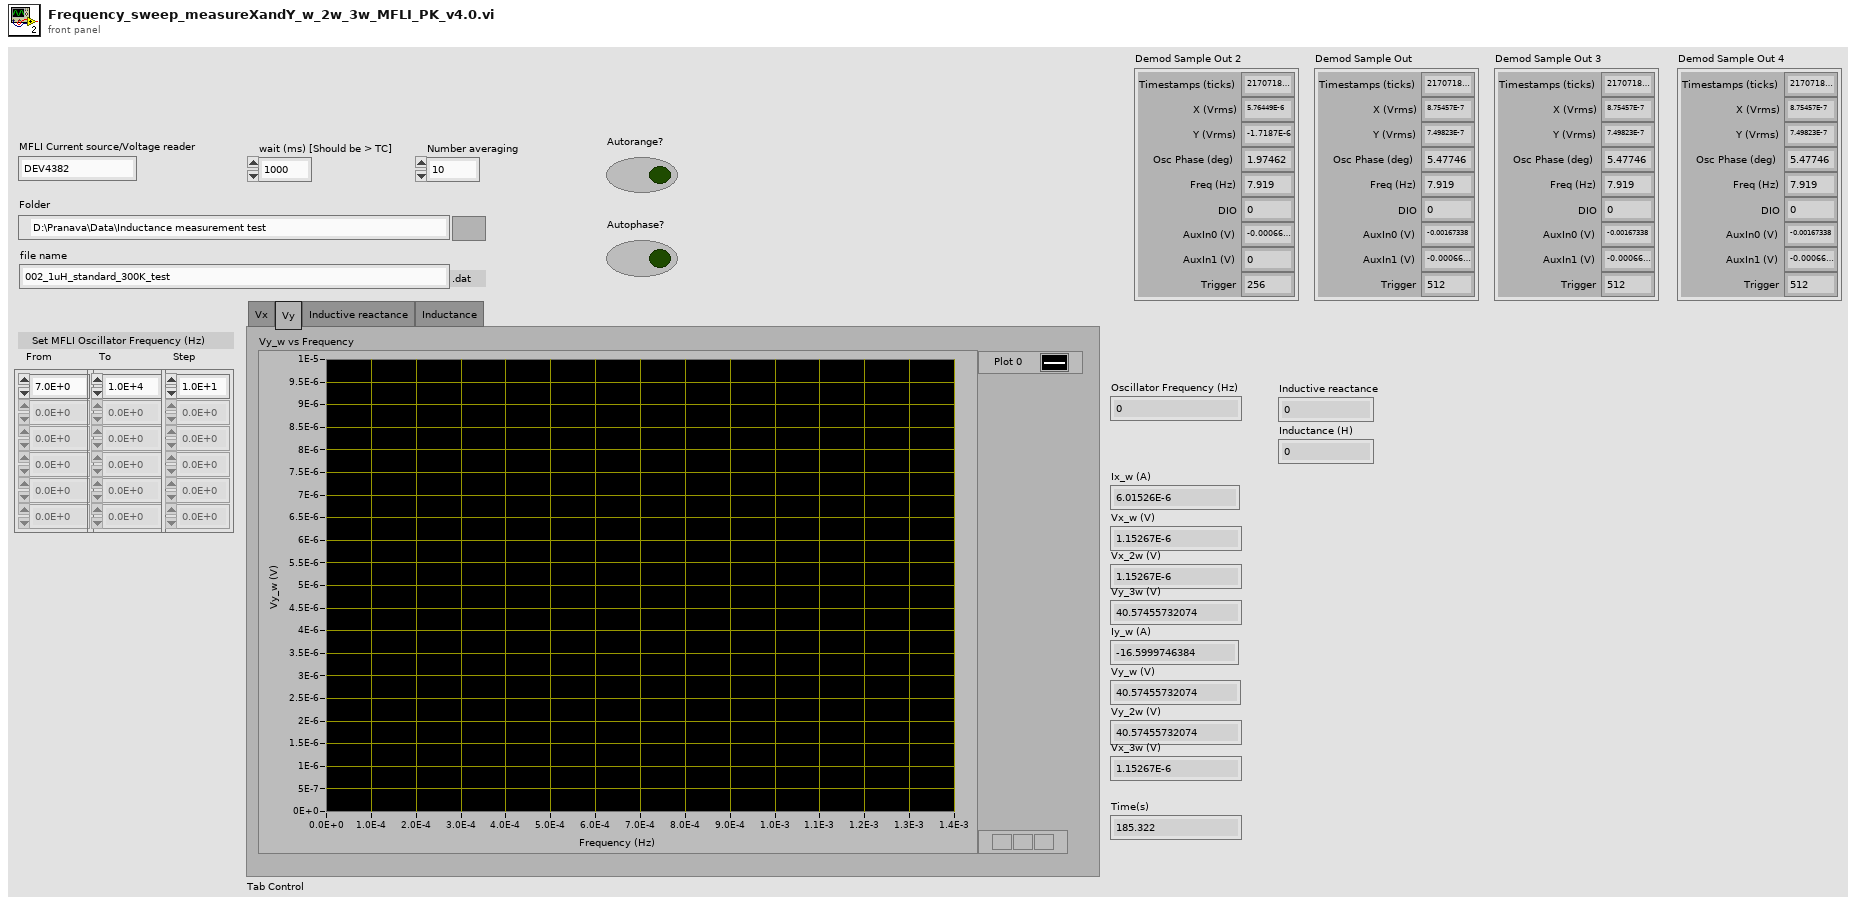
[diagram p1: front panel]
types:
  T1 = enum32{"Vx", "Vy", "Inductive reactance", "Inductance"}
  T2 = typedef "Zurich Instruments LabOne.lvlib/ziTypeDemodSampleSingle.ctl" = cluster{"Timestamps (ticks)":u64, "X (Vrms)":dbl, "Y (Vrms)":dbl, "Osc Phase (deg)":dbl, "Freq (Hz)":dbl, "DIO":u32, "AuxIn0 (V)":dbl, "AuxIn1 (V)":dbl, "Trigger":u32}
  T3 = enum16{"open", "replace", "create", "open or create", "replace or create", "replace or create with confirmation"}
  T4 = typedef "Zurich Instruments LabOne.lvlib/ziTypeHandle.ctl" = cluster{"handleValid":bool, "Conn":u64, "Path Prefix":string, "Handle":u64, "Connected":bool, "Clockbase(s)":dbl}
  T5 = cluster{"Oscillator Frequency (Hz)":dbl, "Vy_w (V)":dbl}
  T6 = cluster{"Oscillator Frequency (Hz)":dbl, "Vx_w (V)":dbl}
  T7 = cluster{"Oscillator Frequency (Hz)":dbl, "Vy_w (V)":dbl}[]
  T8 = cluster{"Oscillator Frequency (Hz)":dbl, "Vx_w (V)":dbl}[]
  T9 = cluster{"Oscillator Frequency (Hz)":dbl, "Field Reading":dbl}[]
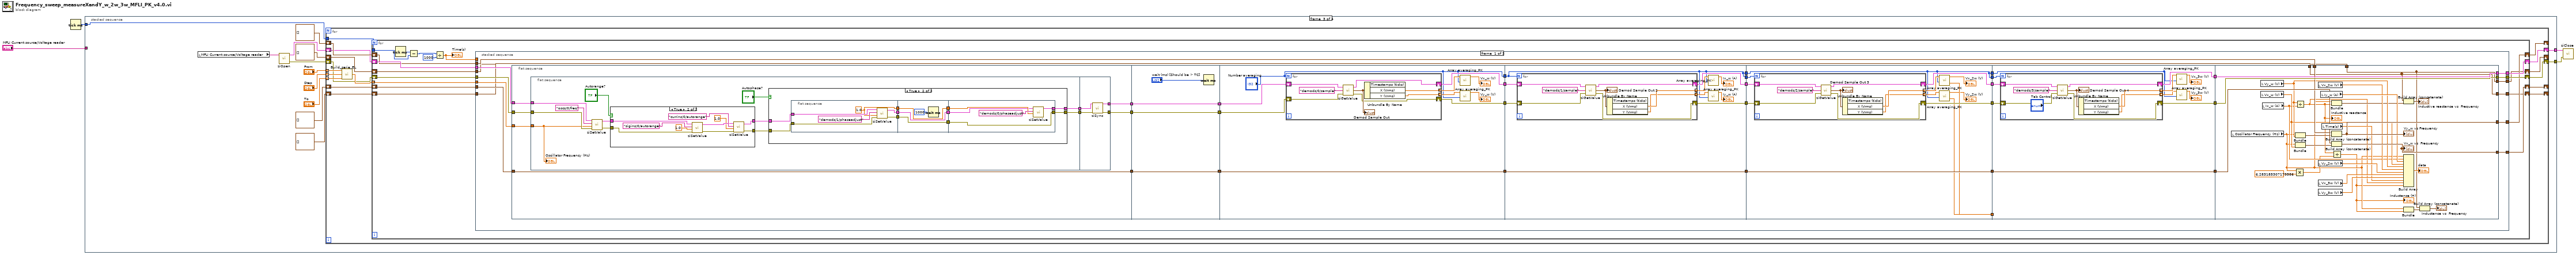
[diagram p0: block diagram]
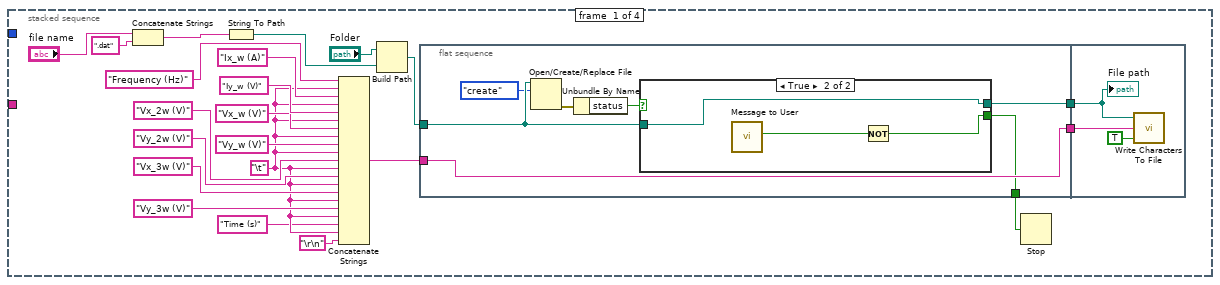
[diagram p2: hidden frame]
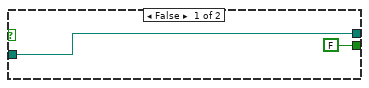
[diagram p3: hidden frame]
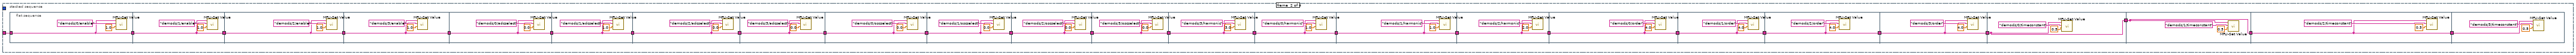
[diagram p4: hidden frame]
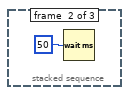
[diagram p7: hidden frame]
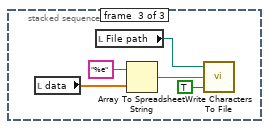
[diagram p8: hidden frame]
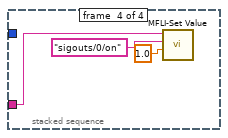
[diagram p9: hidden frame]
diagram:
  n1 = Tick Count (ms)() -> (millisecond timer value=w3:u32)
  n2 = stacked-sequence {
    tunnel: "MFLI Current source/Voltage reader" -> [_ w65 _ w400]
    tunnel: w3 -> [_ _ w146 _]
    tunnel: [_ _ w144 _] -> w2
    tunnel: [_ _ w143 _] -> w1
    frame #0 {
      w6 = "\t"
      n3 = Concatenate Strings("file name", ".dat" ("string")) -> (w23:string)
      n4 = String To Path(string=w23) -> (path=w16:path)
      n5 = Concatenate Strings("Frequency (Hz)" ("string"), w6, "Ix_w (A)" ("string"), w6, "Iy_w (V)" ("string"), w6, "Vx_w (V)" ("string"), w6, "Vy_w (V)" ("string"), w6, "Vx_2w (V)", w6, "Vy_2w (V)", w6, "Vx_3w (V)", w6, "Vy_3w (V)", w6, "Time (s)", w6, "\r\n") -> (w24:string)
      n6 = Build Path(base path="Folder", name or relative path=w16) -> (appended path=w15:path)
      n7 = flat-sequence {
        tunnel: w15 -> [w30]
        tunnel: w24 -> [w33]
        tunnel: [w33] -> w26
        tunnel: [w32] -> w21
        tunnel: [w31] -> w25
        tunnel: w26 -> [w40]
        tunnel: w25 -> [w39]
        frame #0 {
          n8 = Open/Create/Replace File(file path (use dialog)=w30, operation (0:open)=T3."create") -> (error out=w29:errorcluster)  [unwired: 4 in, 2 out]
          n9 = Unbundle By Name(w29) -> ("status"=w27:bool)
          n10 = case shown="True" w27 {
            tunnel: [FALSE ("Yes") w37] -> w32
            tunnel: [w34 w36] -> w31
            tunnel: w30 -> [w34 w36]
            frame False {
            }
            frame True {
              n11 = call "Message to User"() -> ("Yes"=w38:bool)  [unwired: 10 in, 1 out]
              n12 = Not(x=w38) -> (.not. x?=w37:bool)
            }
          }
        }
        frame #1 {
          n13 = call <vilib>:"Write Characters To File.vi"("append to file? (new file:F)"=TRUE, "character string"=w40, "file path (dialog if empty)"=w39) -> ()  [unwired: 2 in, 1 out]
          "File path" <- w39
        }
      }
      n14 = Stop(stop? (T)=w21) -> ()
    }
    frame #1 {
      n15 = flat-sequence {
        tunnel: w65 -> [w66]
        tunnel: [w66] -> w53
        tunnel: w53 -> [w69]
        tunnel: [w69] -> w52
        tunnel: w52 -> [w72]
        tunnel: [w72] -> w51
        tunnel: w51 -> [w75]
        tunnel: [w75] -> w50
        tunnel: [w78] -> w64
        tunnel: w50 -> [w78]
        tunnel: w64 -> [w81]
        tunnel: [w81] -> w63
        tunnel: w63 -> [w84]
        tunnel: [w84] -> w62
        tunnel: w62 -> [w87]
        tunnel: [w87] -> w61
        tunnel: w61 -> [w90]
        tunnel: [w90] -> w60
        tunnel: w60 -> [w93]
        tunnel: [w93] -> w59
        tunnel: w59 -> [w96]
        tunnel: [w96] -> w58
        tunnel: w58 -> [w99]
        tunnel: [w99] -> w57
        tunnel: w57 -> [w102]
        tunnel: [w102] -> w56
        tunnel: w56 -> [w105]
        tunnel: [w105] -> w55
        tunnel: w55 -> [w108]
        tunnel: [w108] -> w54
        tunnel: w54 -> [w111]
        tunnel: [w111] -> w49
        tunnel: w49 -> [w114]
        tunnel: [w114] -> w48
        tunnel: w48 -> [w117]
        tunnel: [w117] -> w47
        tunnel: w47 -> [w120]
        tunnel: [w120] -> w46
        tunnel: w46 -> [w123]
        tunnel: [w123] -> w45
        tunnel: w45 -> [w126]
        tunnel: [w126] -> w44
        tunnel: w44 -> [w129]
        tunnel: [w129] -> w43
        tunnel: w43 -> [w132]
        tunnel: [w132] -> w42
        tunnel: w42 -> [w135]
        frame #0 {
          n16 = call "MFLI-Set Value.vi"("Value"=1.0, "Path"="demods/0/enable", "MFLI Current source/Voltage reader"=w66) -> ()  [unwired: 9 in]
        }
        frame #1 {
          n17 = call "MFLI-Set Value.vi"("Value"=1.0, "Path"="demods/1/enable", "MFLI Current source/Voltage reader"=w69) -> ()  [unwired: 9 in]
        }
        frame #2 {
          n18 = call "MFLI-Set Value.vi"("Value"=1.0, "Path"="demods/2/enable", "MFLI Current source/Voltage reader"=w72) -> ()  [unwired: 9 in]
        }
        frame #3 {
          n19 = call "MFLI-Set Value.vi"("Value"=1.0, "Path"="demods/3/enable", "MFLI Current source/Voltage reader"=w75) -> ()  [unwired: 9 in]
        }
        frame #4 {
          n20 = call "MFLI-Set Value.vi"("Value"=0.0, "Path"="demods/0/adcselect", "MFLI Current source/Voltage reader"=w78) -> ()  [unwired: 9 in]
        }
        frame #5 {
          n21 = call "MFLI-Set Value.vi"("Value"=1.0, "Path"="demods/1/adcselect", "MFLI Current source/Voltage reader"=w81) -> ()  [unwired: 9 in]
        }
        frame #6 {
          n22 = call "MFLI-Set Value.vi"("Value"=0.0, "Path"="demods/2/adcselect", "MFLI Current source/Voltage reader"=w84) -> ()  [unwired: 9 in]
        }
        frame #7 {
          n23 = call "MFLI-Set Value.vi"("Value"=0.0, "Path"="demods/3/adcselect", "MFLI Current source/Voltage reader"=w87) -> ()  [unwired: 9 in]
        }
        frame #8 {
          n24 = call "MFLI-Set Value.vi"("Value"=0.0, "Path"="demods/0/oscselect", "MFLI Current source/Voltage reader"=w90) -> ()  [unwired: 9 in]
        }
        frame #9 {
          n25 = call "MFLI-Set Value.vi"("Value"=0.0, "Path"="demods/1/oscselect", "MFLI Current source/Voltage reader"=w93) -> ()  [unwired: 9 in]
        }
        frame #10 {
          n26 = call "MFLI-Set Value.vi"("Value"=0.0, "Path"="demods/2/oscselect", "MFLI Current source/Voltage reader"=w96) -> ()  [unwired: 9 in]
        }
        frame #11 {
          n27 = call "MFLI-Set Value.vi"("Value"=0.0, "Path"="demods/3/oscselect", "MFLI Current source/Voltage reader"=w99) -> ()  [unwired: 9 in]
        }
        frame #12 {
          n28 = call "MFLI-Set Value.vi"("Value"=3.0, "Path"="demods/3/harmonic", "MFLI Current source/Voltage reader"=w102) -> ()  [unwired: 9 in]
        }
        frame #13 {
          n29 = call "MFLI-Set Value.vi"("Value"=1.0, "Path"="demods/0/harmonic", "MFLI Current source/Voltage reader"=w105) -> ()  [unwired: 9 in]
        }
        frame #14 {
          n30 = call "MFLI-Set Value.vi"("Value"=1.0, "Path"="demods/1/harmonic", "MFLI Current source/Voltage reader"=w108) -> ()  [unwired: 9 in]
        }
        frame #15 {
          n31 = call "MFLI-Set Value.vi"("Value"=2.0, "Path"="demods/2/harmonic", "MFLI Current source/Voltage reader"=w111) -> ()  [unwired: 9 in]
        }
        frame #16 {
          n32 = call "MFLI-Set Value.vi"("Value"=4.0, "Path"="demods/0/order", "MFLI Current source/Voltage reader"=w114) -> ()  [unwired: 9 in]
        }
        frame #17 {
          n33 = call "MFLI-Set Value.vi"("Value"=4.0, "Path"="demods/1/order", "MFLI Current source/Voltage reader"=w117) -> ()  [unwired: 9 in]
        }
        frame #18 {
          n34 = call "MFLI-Set Value.vi"("Value"=4.0, "Path"="demods/2/order", "MFLI Current source/Voltage reader"=w120) -> ()  [unwired: 9 in]
        }
        frame #19 {
          n35 = call "MFLI-Set Value.vi"("Value"=4.0, "Path"="demods/3/order", "MFLI Current source/Voltage reader"=w123) -> ()  [unwired: 9 in]
        }
        frame #20 {
          n36 = call "MFLI-Set Value.vi"("Value"=0.5, "Path"="demods/0/timeconstant", "MFLI Current source/Voltage reader"=w126) -> ()  [unwired: 9 in]
        }
        frame #21 {
          n37 = call "MFLI-Set Value.vi"("Value"=0.5, "Path"="demods/1/timeconstant", "MFLI Current source/Voltage reader"=w129) -> ()  [unwired: 9 in]
        }
        frame #22 {
          n38 = call "MFLI-Set Value.vi"("Value"=0.5, "Path"="demods/2/timeconstant", "MFLI Current source/Voltage reader"=w132) -> ()  [unwired: 9 in]
        }
        frame #23 {
          n39 = call "MFLI-Set Value.vi"("Value"=0.5, "Path"="demods/3/timeconstant", "MFLI Current source/Voltage reader"=w135) -> ()  [unwired: 9 in]
        }
      }
    }
    frame #2 {
      n40 = local read "MFLI Current source/Voltage reader"() -> (w142:string)
      n41 = call "ziOpen.vi"("Address"=w142) -> ("Error Out"=w140:errorcluster, "HandleOut"=w141:T4)  [unwired: 3 in, 1 out]
      n42 = for {
        tunnel: "From" -> [w164] mode=indexing
        tunnel: "To" -> [w163] mode=indexing
        tunnel: "Step" -> [w162] mode=indexing
        shift-right: [w166] -> _
        shift-left: cluster{dbl, "Field Reading":dbl}[] [] -> [w167]
        tunnel: w146 -> [w161]
        shift-right: [w160] -> _
        shift-left: cluster{dbl, "Field Reading":dbl}[] [] -> [w159]
        shift-right: [w158] -> w144
        shift-left: w141 -> [w156]
        shift-right: [w157] -> w143
        shift-left: w140 -> [w155]
        shift-right: [w152] -> _
        shift-left: cluster{dbl, "Field Reading":dbl}[] [] -> [w154]
        shift-right: [w151] -> _
        shift-left: cluster{dbl, "Field Reading":dbl}[] [] -> [w153]
        n43 = call "Build_serie_EL.vi"("end value"=w163, "increment"=w162, "start value"=w164) -> ("output array"=w165:dbl[])
        n44 = for {
          tunnel: w165 -> [w185] mode=indexing
          shift-right: [w183] -> w166
          shift-left: w167 -> [w184]
          shift-right: [w180] -> w158
          shift-left: w156 -> [w182]
          shift-right: [w179] -> w157
          shift-left: w155 -> [w181]
          tunnel: w161 -> [w175]
          shift-right: [w173] -> w160
          shift-left: w159 -> [w172]
          shift-right: [w170] -> w152
          shift-left: w154 -> [w171]
          shift-right: [w168] -> w151
          shift-left: w153 -> [w169]
          n45 = Tick Count (ms)() -> (millisecond timer value=w176:u32)
          n46 = Subtract(x=w176, y=w175) -> (x-y=w177:u32)
          n47 = Divide(x=w177, y=1000) -> (x/y=w174:dbl)
          "Time(s)" <- w174
          n48 = stacked-sequence {
            tunnel: w185 -> [w221 _ _]
            tunnel: w184 -> [w222 _ _]
            tunnel: [w223 _ _] -> w183
            tunnel: w182 -> [w214 _ _]
            tunnel: w181 -> [w213 _ _]
            tunnel: [w209 _ _] -> w180
            tunnel: [w208 _ _] -> w179
            tunnel: w174 -> [_ _ _]
            tunnel: [w191 _ _] -> w173
            tunnel: w172 -> [w190 _ _]
            tunnel: w171 -> [w189 _ _]
            tunnel: [w188 _ _] -> w170
            tunnel: w169 -> [w187 _ _]
            tunnel: [w186 _ _] -> w168
            frame #0 {
              n49 = flat-sequence {
                tunnel: [w231] -> w219
                tunnel: w221 -> [w229]
                tunnel: w222 -> [w231]
                tunnel: [w224] -> w216
                tunnel: [w225] -> w215
                tunnel: w214 -> [w230]
                tunnel: w213 -> [w228]
                tunnel: w219 -> [w290]
                tunnel: [w290] -> w220
                tunnel: [w288] -> w218
                tunnel: [w287] -> w217
                tunnel: w216 -> [w287]
                tunnel: w215 -> [w288]
                tunnel: [w300] -> w212
                tunnel: w217 -> [w299]
                tunnel: w218 -> [w298]
                tunnel: w220 -> [w300]
                tunnel: [w297] -> w211
                tunnel: [w296] -> w210
                tunnel: ["Number averaging"] -> w200
                tunnel: w212 -> [w318]
                tunnel: [w318] -> w207
                tunnel: w211 -> [w317]
                tunnel: w210 -> [w316]
                tunnel: [w315] -> w206
                tunnel: [w314] -> w205
                tunnel: w200 -> [w310]
                tunnel: [w310] -> w198
                tunnel: [w310] -> w197
                tunnel: w207 -> [w337]
                tunnel: [w337] -> w204
                tunnel: w206 -> [w336]
                tunnel: w205 -> [w335]
                tunnel: [w331] -> w202
                tunnel: [w332] -> w199
                tunnel: w198 -> [w330]
                tunnel: w197 -> [w329]
                tunnel: [w329] -> w195
                tunnel: [w329] -> w194
                tunnel: [w328] -> w193
                tunnel: [w327] -> w192
                tunnel: w204 -> [w356]
                tunnel: [w356] -> w203
                tunnel: w202 -> [w354]
                tunnel: [w352] -> w201
                tunnel: w199 -> [w355]
                tunnel: [w353] -> w196
                tunnel: w195 -> [w349]
                tunnel: w194 -> [w348]
                tunnel: w193 -> [_]
                tunnel: w192 -> [_]
                tunnel: [w393] -> w223
                tunnel: w203 -> [w392]
                tunnel: [w391] -> w209
                tunnel: [w390] -> w208
                tunnel: w201 -> [w390]
                tunnel: w196 -> [w391]
                tunnel: [w389] -> w191
                tunnel: w190 -> [w388]
                tunnel: w189 -> [w368]
                tunnel: [w368] -> w188
                tunnel: w187 -> [w365]
                tunnel: [w365] -> w186
                frame #0 {
                  n50 = flat-sequence {
                    tunnel: w230 -> [w240]
                    tunnel: w229 -> [w232]
                    tunnel: w228 -> [w239]
                    tunnel: [w238] -> w227
                    tunnel: [w237] -> w226
                    tunnel: [w286] -> w225
                    tunnel: [w285] -> w224
                    tunnel: w226 -> [w283]
                    tunnel: w227 -> [w284]
                    frame #0 {
                      n51 = call-poly "ziSetValue.vi"("Error In"=w239, "Value"=w232, "Path"="oscs/0/freq", "Handle In"=w240) -> ("Error Out"=w241:errorcluster, "Handle Out"=w242:T4)  [unwired: 1 in]
                      n52 = case shown="True" "Autorange?" {
                        tunnel: w242 -> [w271 w282]
                        tunnel: w241 -> [w272 w279]
                        tunnel: [w272 w274] -> w236
                        tunnel: [w271 w273] -> w235
                        frame False {
                        }
                        frame True {
                          n53 = call-poly "ziSetValue.vi"("Error In"=w279, "Value"=1.0, "Path"="sigins/0/autorange", "Handle In"=w282) -> ("Error Out"=w276:errorcluster, "Handle Out"=w277:T4)  [unwired: 1 in]
                          n54 = call-poly "ziSetValue.vi"("Error In"=w276, "Value"=1.0, "Path"="currins/0/autorange", "Handle In"=w277) -> ("Error Out"=w274:errorcluster, "Handle Out"=w273:T4)  [unwired: 1 in]
                        }
                      }
                      n55 = case shown="True" "Autophase?" {
                        tunnel: [w245 w255] -> w238
                        tunnel: [w244 w254] -> w237
                        tunnel: w236 -> [w244 w253]
                        tunnel: w235 -> [w245 w252]
                        frame False {
                        }
                        frame True {
                          n56 = flat-sequence {
                            tunnel: w253 -> [w259]
                            tunnel: w252 -> [w257]
                            tunnel: [w261] -> w251
                            tunnel: [w260] -> w250
                            tunnel: [w256] -> w246
                            tunnel: w251 -> [w265]
                            tunnel: w250 -> [w264]
                            tunnel: [w265] -> w249
                            tunnel: [w264] -> w248
                            tunnel: [w262] -> w247
                            tunnel: w246 -> [w262]
                            tunnel: [w270] -> w254
                            tunnel: [w266] -> w255
                            tunnel: w249 -> [w267]
                            tunnel: w248 -> [w270]
                            tunnel: w247 -> [w268]
                            frame #0 {
                              w256 = 1.0
                              n57 = call-poly "ziSetValue.vi"("Error In"=w259, "Value"=w256, "Path"="demods/1/phaseadjust", "Handle In"=w257) -> ("Error Out"=w260:errorcluster, "Handle Out"=w261:T4)  [unwired: 1 in]
                            }
                            frame #1 {
                              n58 = Wait (ms)(milliseconds to wait=1000) -> ()  [unwired: 1 out]
                            }
                            frame #2 {
                              n59 = call-poly "ziSetValue.vi"("Value"=w268, "Path"="demods/0/phaseadjust", "Handle In"=w267) -> ("Handle Out"=w266:T4)  [unwired: 2 in, 1 out]
                            }
                          }
                        }
                      }
                      "Oscillator Frequency (Hz)" <- w232
                    }
                    frame #1 {
                      n60 = call "ziSync.vi"("Handle In"=w284, "Error In"=w283) -> ("Handle Out"=w286:T4, "Error Out"=w285:errorcluster)  [unwired: 12 in]
                    }
                  }
                }
                frame #1 {
                  n61 = Wait (ms)(milliseconds to wait="wait (ms) [Should be > TC]") -> ()  [unwired: 1 out]
                }
                frame #2 {
                  n62 = for {
                    N: "Number averaging" -> [_]
                    tunnel: [w302] -> w294 mode=indexing
                    tunnel: [w301] -> w293 mode=indexing
                    shift-right: [w303] -> w296
                    shift-left: w299 -> [w306]
                    shift-right: [w304] -> w297
                    shift-left: w298 -> [w305]
                    n63 = call-poly "ziGetValue.vi"("error in"=w306, "Path"="demods/0/sample", "Handle In"=w305) -> ("error out"=w303:errorcluster, "Demod Sample Out"=w307:T2, "Handle Out"=w304:T4)
                    "Demod Sample Out" <- w307
                    n64 = Unbundle By Name(w307) -> ("X (Vrms)"=w302:dbl, "Y (Vrms)"=w301:dbl)  [unwired: 1 out]
                  }
                  n65 = call "Array averaging_PK.vi"("Number averaging"="Number averaging", "numeric array"=w294) -> ("Average value"=→"Vx_w (V)":dbl)  [unwired: 9 in]
                  n66 = call "Array averaging_PK.vi"("Number averaging"="Number averaging", "numeric array"=w293) -> ("Average value"=→"Vy_w (V)":dbl)  [unwired: 9 in]
                }
                frame #3 {
                  n67 = for {
                    N: w310 -> [_]
                    tunnel: [w320] -> w312 mode=indexing
                    tunnel: [w319] -> w311 mode=indexing
                    shift-right: [w322] -> w315
                    shift-left: w317 -> [w324]
                    shift-right: [w321] -> w314
                    shift-left: w316 -> [w323]
                    n68 = call-poly "ziGetValue.vi"("error in"=w323, "Path"="demods/1/sample", "Handle In"=w324) -> ("error out"=w321:errorcluster, "Demod Sample Out"=w325:T2, "Handle Out"=w322:T4)
                    "Demod Sample Out 2" <- w325
                    n69 = Unbundle By Name(w325) -> ("X (Vrms)"=w320:dbl, "Y (Vrms)"=w319:dbl)  [unwired: 1 out]
                  }
                  n70 = call "Array averaging_PK.vi"("Number averaging"=w310, "numeric array"=w312) -> ("Average value"=→"Ix_w (A)":dbl)  [unwired: 9 in]
                  n71 = call "Array averaging_PK.vi"("Number averaging"=w310, "numeric array"=w311) -> ("Average value"=→"Iy_w (A)":dbl)  [unwired: 9 in]
                }
                frame #4 {
                  n72 = for {
                    N: w330 -> [_]
                    tunnel: [w339] -> w333 mode=indexing
                    tunnel: [w338] -> w334 mode=indexing
                    shift-right: [w341] -> w332
                    shift-left: w336 -> [w343]
                    shift-right: [w340] -> w331
                    shift-left: w335 -> [w342]
                    n73 = call-poly "ziGetValue.vi"("error in"=w342, "Path"="demods/2/sample", "Handle In"=w343) -> ("error out"=w340:errorcluster, "Demod Sample Out"=w344:T2, "Handle Out"=w341:T4)
                    "Demod Sample Out 3" <- w344
                    n74 = Unbundle By Name(w344) -> ("X (Vrms)"=w339:dbl, "Y (Vrms)"=w338:dbl)  [unwired: 1 out]
                  }
                  n75 = call "Array averaging_PK.vi"("Number averaging"=w329, "numeric array"=w333) -> ("Average value"=w328:dbl)  [unwired: 9 in]
                  "Vx_2w (V)" <- w328
                  n76 = call "Array averaging_PK.vi"("Number averaging"=w329, "numeric array"=w334) -> ("Average value"=w327:dbl)  [unwired: 9 in]
                  "Vy_2w (V)" <- w327
                }
                frame #5 {
                  n77 = for {
                    N: w349 -> [_]
                    tunnel: [w358] -> w351 mode=indexing
                    tunnel: [w357] -> w350 mode=indexing
                    shift-right: [w360] -> w353
                    shift-left: w355 -> [w362]
                    shift-right: [w359] -> w352
                    shift-left: w354 -> [w361]
                    n78 = call-poly "ziGetValue.vi"("error in"=w361, "Path"="demods/3/sample", "Handle In"=w362) -> ("error out"=w359:errorcluster, "Demod Sample Out"=w363:T2, "Handle Out"=w360:T4)
                    "Demod Sample Out 4" <- w363
                    n79 = Unbundle By Name(w363) -> ("X (Vrms)"=w358:dbl, "Y (Vrms)"=w357:dbl)  [unwired: 1 out]
                  }
                  n80 = call "Array averaging_PK.vi"("Number averaging"=w348, "numeric array"=w351) -> ("Average value"=→"Vx_3w (V)":dbl)  [unwired: 9 in]
                  n81 = call "Array averaging_PK.vi"("Number averaging"=w348, "numeric array"=w350) -> ("Average value"=→"Vy_3w (V)":dbl)  [unwired: 9 in]
                }
                frame #6 {
                  n82 = local read "Oscillator Frequency (Hz)"() -> (w367:dbl)
                  n83 = local read "Vy_w (V)"() -> (w377:dbl)
                  n84 = local read "Vx_w (V)"() -> (w378:dbl)
                  n85 = local read "Ix_w (A)"() -> (w376:dbl)
                  n86 = Multiply(x=w367, y=6.283185307179586) -> (x*y=w374:dbl)
                  n87 = Divide(x=w377, y=w376) -> (x/y=w371:dbl)
                  "Inductive reactance" <- w371
                  n88 = Bundle("Oscillator Frequency (Hz)"=w367, "Vy_w (V)"=w377) -> (w386:T5)  [unwired: 1 in]
                  n89 = Bundle("Oscillator Frequency (Hz)"=w367, "Vx_w (V)"=w378) -> (w387:T6)  [unwired: 1 in]
                  n90 = local read "Vx_2w (V)"() -> (w383:dbl)
                  n91 = local read "Vy_2w (V)"() -> (w382:dbl)
                  n92 = local read "Vx_3w (V)"() -> (w381:dbl)
                  n93 = local read "Vy_3w (V)"() -> (w380:dbl)
                  n94 = local read "Iy_w (A)"() -> (w385:dbl)
                  n95 = local read "Time(s)"() -> (w379:dbl)
                  n96 = Bundle("Oscillator Frequency (Hz)"=w367, w371) -> (w373:cluster{"Oscillator Frequency (Hz)":dbl, dbl})  [unwired: 1 in]
                  n97 = Build Array (concatenate)(w388, w386) -> (w389:T7)
                  "Vy_w vs Frequency" <- w389
                  n98 = Build Array (concatenate)(w392, w387) -> (w393:T8)
                  "Vx_w vs  Frequency" <- w393
                  n99 = Divide(x=w371, y=w374) -> (x/y=w366:dbl)
                  "Inductance (H)" <- w366
                  n100 = Build Array (concatenate)(w368, w373) -> (→"Inductive reactance vs  Frequency":T9)
                  n101 = Build Array(w367, w376, w385, w378, w377, w383, w382, w381, w380, w379, w371, w366) -> (→"data":dbl[])
                  n102 = Bundle("Oscillator Frequency (Hz)"=w367, w366) -> (w370:cluster{"Oscillator Frequency (Hz)":dbl, dbl})  [unwired: 1 in]
                  n103 = Build Array (concatenate)(w365, w370) -> (→"Inductance vs  Frequency":T9)
                }
              }
            }
            frame #1 {
              n104 = Wait (ms)(milliseconds to wait=u32 50) -> ()  [unwired: 1 out]
            }
            frame #2 {
              n105 = local read "data"() -> (w395:dbl[])
              n106 = local read "File path"() -> (w397:path)
              n107 = Array To Spreadsheet String(array=w395, 3:"%e" ("format string")) -> (spreadsheet string=w398:string)  [unwired: 1 in]
              n108 = call <vilib>:"Write Characters To File.vi"("append to file? (new file:F)"=TRUE, "character string"=w398, "file path (dialog if empty)"=w397) -> ()  [unwired: 2 in, 1 out]
            }
          }
        }
      }
    }
    frame #3 {
      n109 = call "MFLI-Set Value.vi"("Value"=1.0, "Path"="sigouts/0/on", "MFLI Current source/Voltage reader"=w400) -> ()  [unwired: 9 in]
    }
  }
  n110 = call "ziClose.vi"("Error In"=w1, "Handle In"=w2) -> ()  [unwired: 4 out]
